vi "LogMessage.vi"(9 "Log?":bool=TRUE, 11 "Message":string) -> (2 "Logs":string[](array[string]))   [LabVIEW 2012]
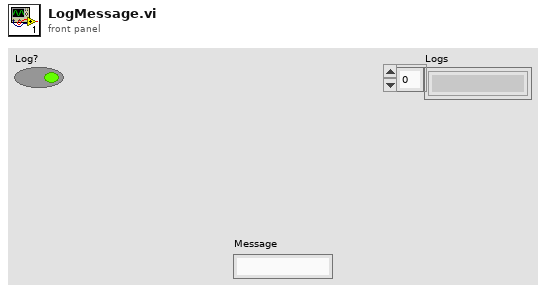
[diagram p1: front panel]
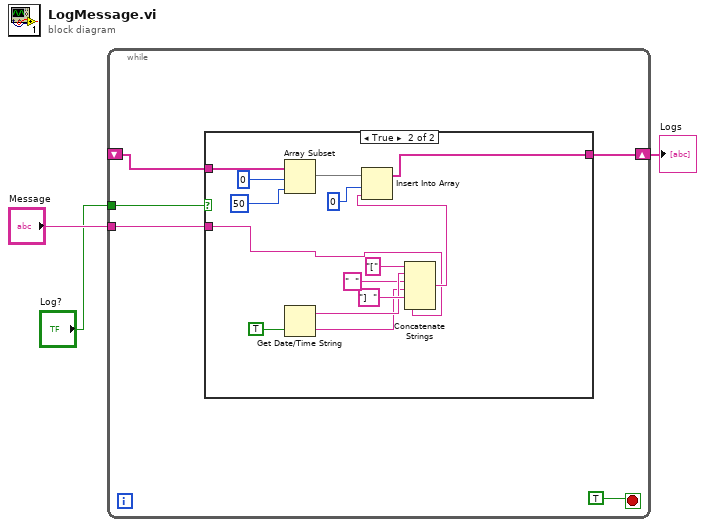
[diagram p0: block diagram]
diagram:
  n1 = while {
    tunnel: "Message" -> [w5]
    shift-right: [w6] -> w1
    shift-left: _ -> [w7]
    tunnel: "Log?" -> [w4]
    stop <- TRUE stop-if-true
    n2 = case shown="True" w4 {
      tunnel: w7 -> [w9 w23]
      tunnel: [w9 w18] -> w6
      tunnel: w5 -> [_ w14]
      frame False {
      }
      frame True {
        n3 = Array Subset(array=w23, index=0, length=50) -> (w20:string[])
        n4 = Get Date/Time String(want seconds? (F)=TRUE) -> (date string=w12:string, time string=w11:string)  [unwired: 2 in]
        n5 = Concatenate Strings("[", w12, "  ", w11, "]  ", w14) -> (w15:string)
        n6 = Insert Into Array(array=w20, index=0, new element=w15) -> (w18:string[])
      }
    }
  }
  "Logs" <- w1
